vi "AnalyseTestRun.vi"() -> ()   [LabVIEW 2024]
panel:
  out "Array":string[](array[string])
  out "size":i64
  out "Test_Finish":timestamp
  out "Test_Start":timestamp
  out "Overall Temperature Stats":string
  in  "Top Directory":path
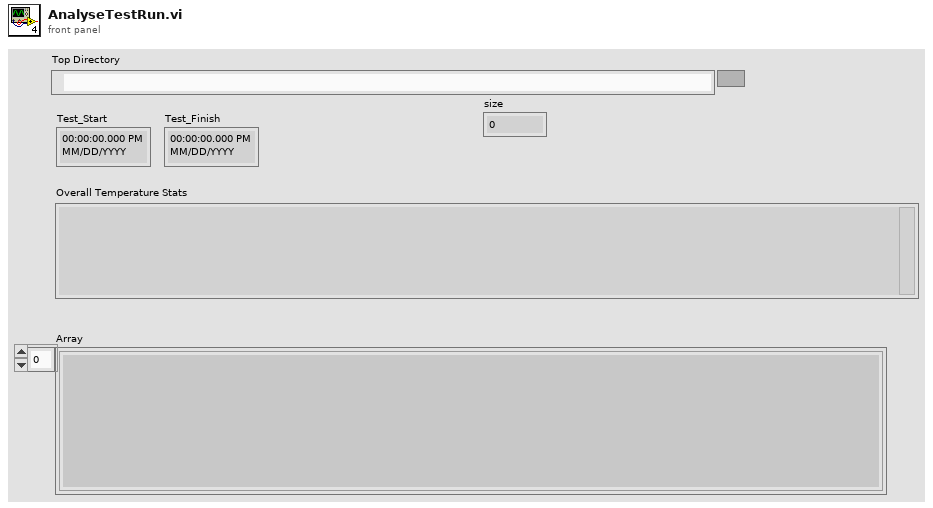
[diagram p1: front panel]
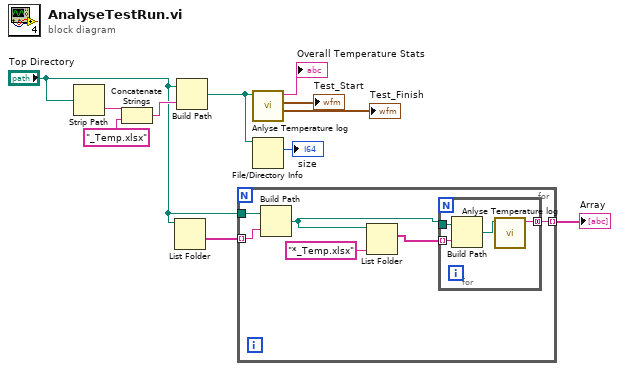
[diagram p0: block diagram]
diagram:
  n1 = Strip Path(path="Top Directory") -> (name=w11:string)  [unwired: 1 out]
  n2 = Concatenate Strings(w11, "_Temp.xlsx" ("string")) -> (w9:string)
  n3 = List Folder(path="Top Directory") -> (folder names=w3:string[])  [unwired: 3 in, 3 out]
  n4 = Build Path(base path="Top Directory", name or relative path=w9) -> (appended path=w4:path)
  n5 = for {
    tunnel: w3 -> [w14] mode=indexing
    tunnel: "Top Directory" -> [w17]
    tunnel: [w16] -> w1 mode=indexing
    n6 = Build Path(base path=w17, name or relative path=w14) -> (appended path=w15:path)
    n7 = List Folder(path=w15, pattern="*_Temp.xlsx" ("string")) -> (filenames=w12:string[])  [unwired: 2 in, 3 out]
    n8 = for {
      tunnel: [w21] -> w16 mode=concatenating
      tunnel: w15 -> [w19]
      tunnel: w12 -> [w18] mode=indexing
      n9 = Build Path(base path=w19, name or relative path=w18) -> (appended path=w20:path)
      n10 = call "Anlyse Temperature log.vi"("Temperature Log File"=w20) -> ("Report"=w21:string)  [unwired: 8 in, 2 out]
    }
  }
  "Array" <- w1
  n11 = call "Anlyse Temperature log.vi"("Temperature Log File"=w4) -> ("Test_Finish"=→"Test_Finish":timestamp, "Test_Start"=→"Test_Start":timestamp, "Report"=→"Overall Temperature Stats":string)  [unwired: 8 in]
  n12 = File/Directory Info(path=w4) -> (size=→"size":i64)  [unwired: 1 in, 6 out]
